vi "ADCP_UI_Event_Structure.vi"(8 "error in (no error)":errorcluster, 11 "ADCU_GUI References":T1) -> ()   [LabVIEW 2017]
uses:
  Controls/ADCP_UI/ADCP_UI_Parameters.ctl
  Controls/ADCP_UI/ADCP_UI_Queues.ctl
  Controls/ADCP_UI/ADCP_UI_Continuous_Receiver_States.ctl
  Controls/ADCP_UI/ADCP_Queue_Receive_Log_Queue_Element.ctl
  Controls/Packet/Packet.ctl
  Controls/Packet/Packet_Direction.ctl
  Controls/Packet/Packet_Type.ctl
  Controls/Packet/Packet_Priority.ctl
  Controls/Data Packets/Data_Packet.ctl
  Controls/Data Packets/Parameter.ctl
  Controls/Data Packets/Parameter_Data_Type.ctl
  Controls/Data Packets/Data_Packet_Transmit_Mode.ctl
  Controls/Data Packets/Data_Packet_FGV_Commands.ctl
  Controls/ADCP_UI/ADCP_UI_Queue_Manager_Commands.ctl
  Controls/Connection Management/Connection_Management_Commands.ctl
  Controls/ADCP_UI/ADCP_UI_Node_Requests.ctl
  ADCP_UI_Receive_List_Data_Packets.vi
panel:
  out "Connect/Disconnect COM Port":bool
  out "Remove transmit list frame":bool
  out "Add transmit list frame":bool
  out "Request frames from node":bool
  out "Add request frame":bool
  out "Remove request frame":bool
  out "Enable / disable node":bool
  out "Get node status":bool
  out "Reset nodes":bool
  out "Reset node":bool
  out "Load Symbol File":bool
  out "Application Stoppped":bool
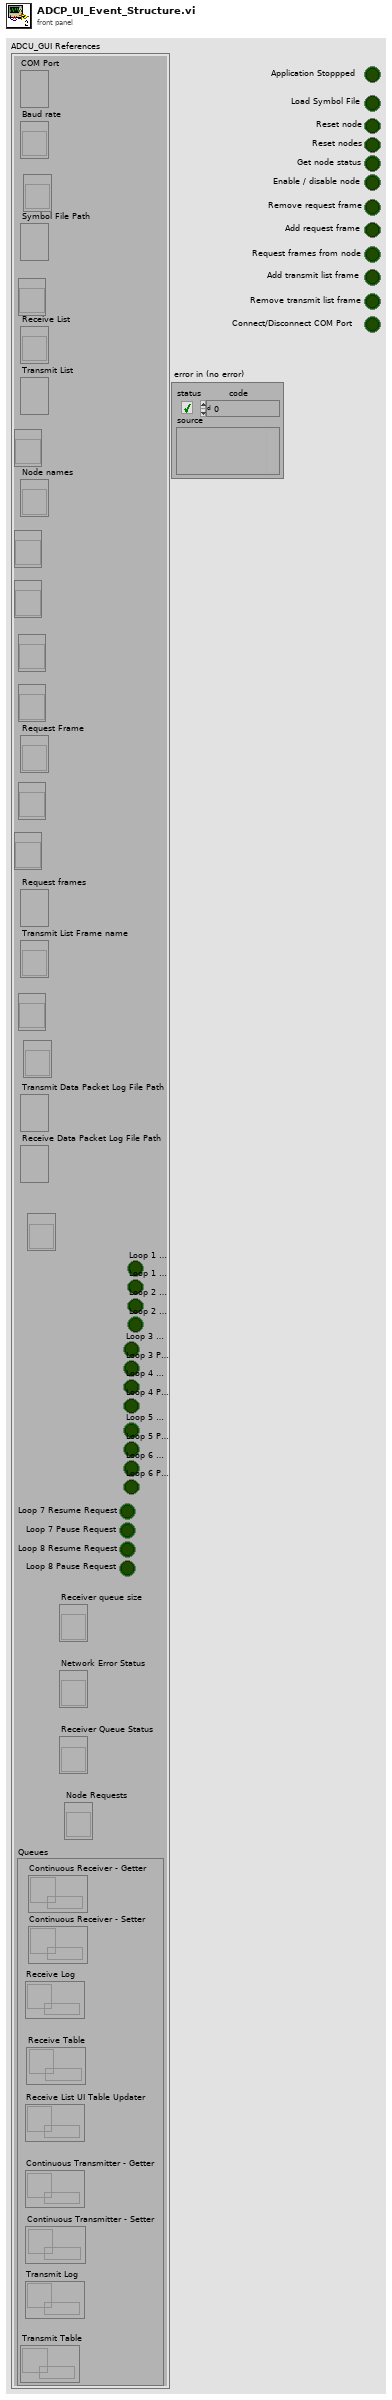
[diagram p1: front panel]
types:
  T1 = typedef "ADCP_UI_Parameters.ctl" = cluster{"COM Port":refnum<vi>, "Baud rate":refnum<vi>, "Symbol File Path":refnum<vi>, "Receive List":refnum<vi>, "Transmit List":refnum<vi>, "Node names":refnum<vi>, "Request Frame":refnum<vi>, "Request frames":refnum<vi>, "Transmit List Frame name":refnum<vi>, "Transmit Data Packet Log File Path":refnum<vi>, "Receive Data Packet Log File Path":refnum<vi>, "Loop 1 Resume Request":bool, "Loop 1 Pause Request":bool, "Loop 2 Resume Request":bool, "Loop 2 Pause Request":bool, "Loop 3 Resume Request":bool, "Loop 3 Pause Request":bool, "Loop 4 Resume Request":bool, "Loop 4 Pause Request":bool, "Loop 5 Resume Request":bool, "Loop 5 Pause Request":bool, "Loop 6 Resume Request":bool, "Loop 6 Pause Request":bool, "Loop 7 Resume Request":bool, "Loop 7 Pause Request":bool, "Loop 8 Resume Request":bool, "Loop 8 Pause Request":bool, "Exit":refnum<vi>, "Connect/Disconnect":refnum<vi>, "Load Symbol File":refnum<vi>, "Reset node":refnum<vi>, "Reset nodes":refnum<vi>, "Get node status":refnum<vi>, "Enable/disable node":refnum<vi>, "Request frames from node":refnum<vi>, "Remove request frame":refnum<vi>, "Add request frame":refnum<vi>, "Remove transmit list frame":refnum<vi>, "Add transmit list frame":refnum<vi>, "Receiver queue size":refnum<vi>, "Network Error Status":refnum<vi>, "Receiver Queue Status":refnum<vi>, "Node Requests":refnum<vi>, "Queues":T2}
  T2 = typedef "ADCP_UI_Queues.ctl" = cluster{"Continuous Receiver - Getter":refnum<queue>, "Continuous Receiver - Setter":refnum<queue>, "Receive Log":refnum<queue>, "Receive Table":refnum<queue>, "Receive List UI Table Updater":refnum<queue>, "Continuous Transmitter - Getter":refnum<queue>, "Continuous Transmitter - Setter":refnum<queue>, "Transmit Log":refnum<queue>, "Transmit Table":refnum<queue>}
  T3 = typedef "Data_Packet_FGV_Commands.ctl" = enum16{"Update all parameters from data packets", "Update Packet", "Load", "Read Packet Parameters", "Write Packet Parameters", "Read Packet Parameter", "Write Packet Parameter", "Read Data Packets", "Read Data Packet", "Read Data Packet by Parameter Name", "Get Parameter Node and Frame ID", "Read Data Packet from Node ID and Frame ID"}
  T4 = typedef "ADCP_UI_Queue_Manager_Commands.ctl" = enum16{"Disable Continuous Receiver", "Enable Continuous Receiver", "Disable Continuous Transmitter", "Enable Continuous Transmitter", "Enable Continuous Tx & Rx", "Disable Continuous Tx & Rx"}
  T5 = typedef "ADCP_UI_Node_Requests.ctl" = enum16{"None", "Open Connection RQST", "Open Connection ACK", "Close Connection RQST", "Close Connection ACK", "Sync/Reset RQST", "Sync/Reset ACK", "Error & Status RQST", "Error & Status ACK", "Remote Request RQST", "Remote Request ACK", "Timeout"}
  T6 = typedef "Connection_Management_Commands.ctl" = enum16{"Sync/Reset", "Open Connection", "Close Connection"}
  T7 = typedef "Packet.ctl" = cluster{"Raw Bytes":u8[], "Checksum":bool, "Direction":T8, "Processed Bytes":u8[], "Node ID":u8, "Packet type":T9, "Frame Data":u32, "Priority":T10, "Frame ID":u8}
  T8 = typedef "Packet_Direction.ctl" = enum16{"Transmit", "Receive", "Bidirectional"}
  T9 = typedef "Packet_Type.ctl" = enum16{"Data", "Connection Management", "Remote Request", "Error/Status"}
  T10 = typedef "Packet_Priority.ctl" = enum16{"LOW", "HIGH"}
  T11 = typedef "Data_Packet_Transmit_Mode.ctl" = enum16{"Disabled", "Single", "Cyclic"}
  T12 = typedef "Parameter.ctl" = cluster{"Parameter name":string, "Node name":string, "Node ID":u8, "Frame name":string, "Frame ID":u8, "Data type":T13, "Start Bit":i32, "Bit Length":i32, "Factor":dbl, "Offset":dbl, "Minimum":dbl, "Maximum":dbl, "Descriptor":string, "Enum values":string[], "Value":string}
  T13 = typedef "Parameter_Data_Type.ctl" = enum16{"BOOL", "UNSIGNED", "SIGNED", "FLOAT32", "ENUM"}
  T14 = typedef "LVComboBoxStrsAndValuesArrayTypeDef.ctl" = cluster{"String":string, "Value":string}[]
  T15 = typedef "CM_Param.ctl" = cluster{"Sync/Reset RQST":bool, "Sync/Reset ACK":bool, "Open Conn. RQST":bool, "Open Conn. ACK":bool, "Close Conn. RQST":bool, "Close Conn. ACK":bool}
  T16 = typedef "ES_Param.ctl" = cluster{"Status Request":bool, "Status Ack.":bool, "Receiver Queue Status":enum16{"OK", "EMPTY", "FULL"}, "Network Error Status":enum16{"NONE", "CONNECTION_ALREADY_OPEN", "CONNECTION_ALREADY_CLOSED", "INVALID_FRAME_REQUEST"}, "Application Error Code":u16, "Receiver Queue Size":i32}
  T17 = enum16{"NONE", "CONNECTION_ALREADY_OPEN", "CONNECTION_ALREADY_CLOSED", "INVALID_FRAME_REQUEST"}
  T18 = typedef "RREQ_Param.ctl" = cluster{"Remote Request":bool, "Remote Ack.":bool, "Number of frames":u8, "FID_0":u8, "FID_1":u8, "FID_2":u8, "FID_3":u8}
  T19 = typedef "ADCP_UI_Data_Packet_Receiver_Parameters.ctl" = cluster{"Node ID":u32, "Frame ID":u32, "Count":u32, "Last received time (ms)":u32, "Time interval (ms)":u32}
  T20 = typedef "Data_Packet.ctl" = cluster{"Packet":T7, "Parameters":T12[], "Last Received Time (ms)":u64, "Receive count":i32, "Transmit count":i32, "Transmit interval (ms)":u32, "Last Transmitted Time (ms)":u64, "Receive interval (ms)":u32, "Transmit_Mode":T11, "Transmit Enable":bool, "Cyclic Transmit interval (ms)":u32}
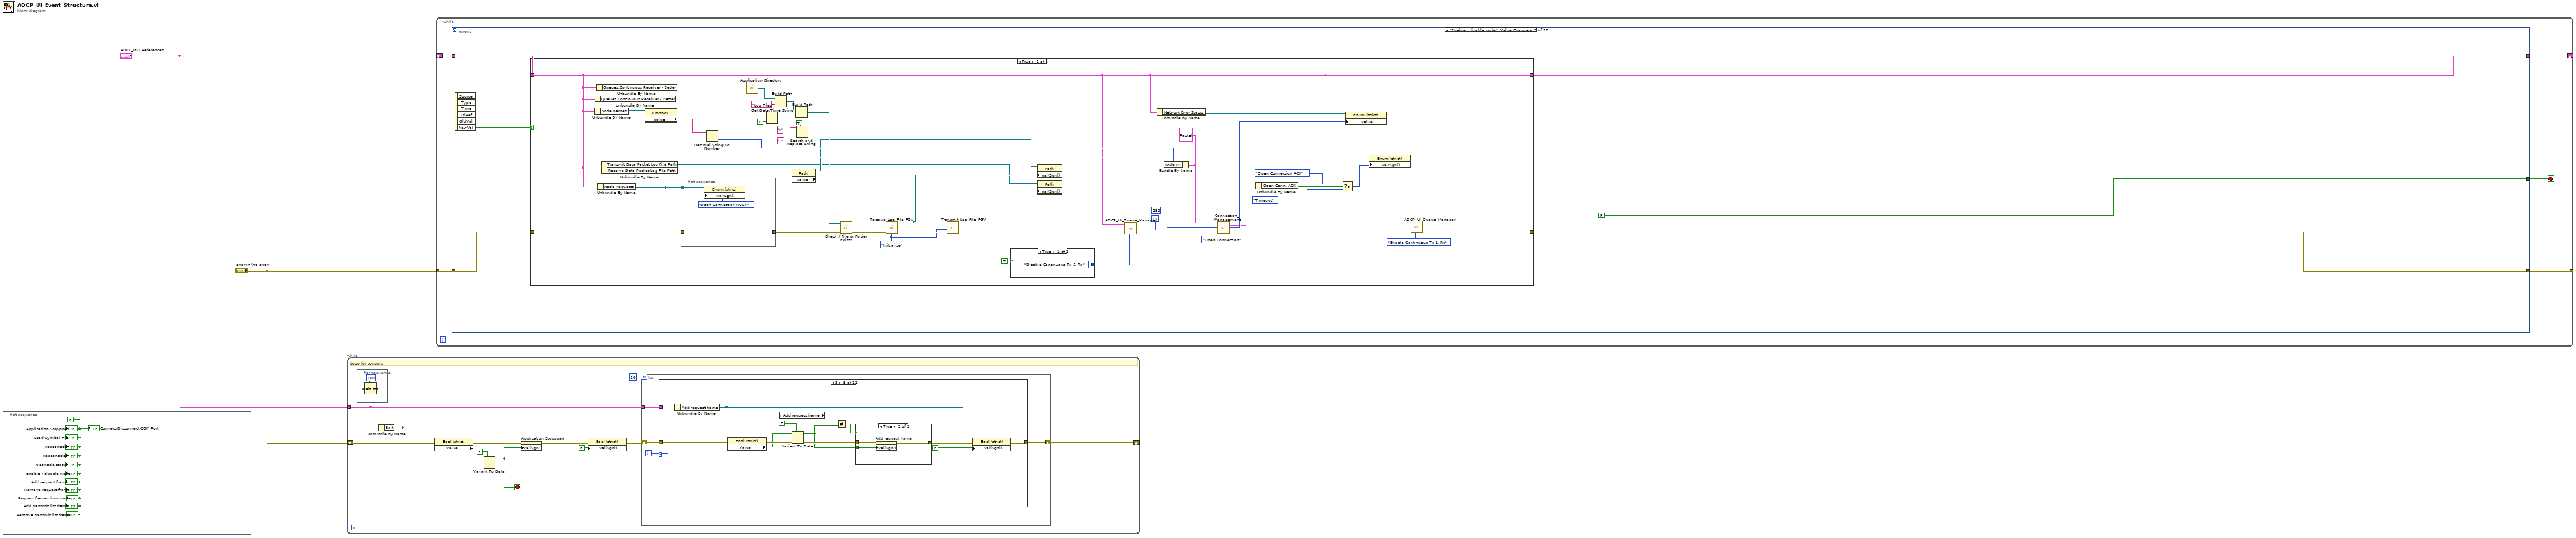
[diagram p0: block diagram]
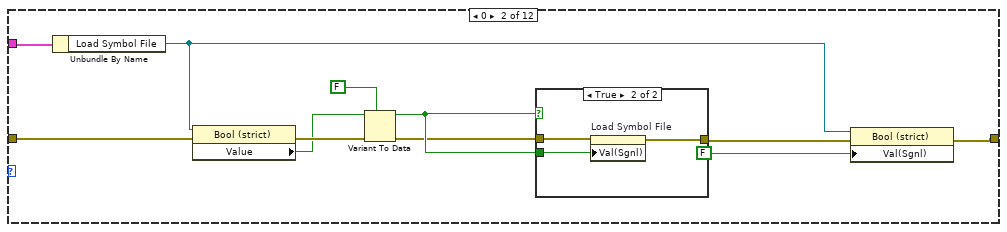
[diagram p3: hidden frame]
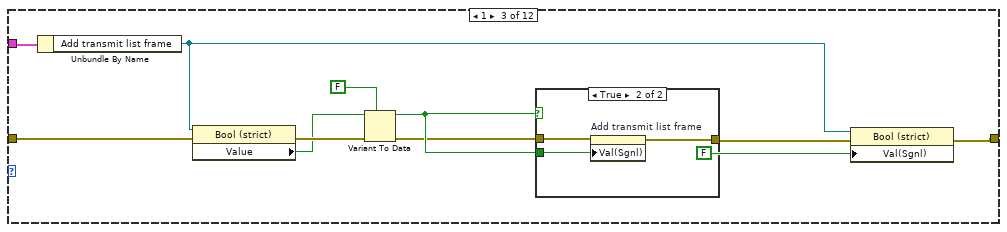
[diagram p5: hidden frame]
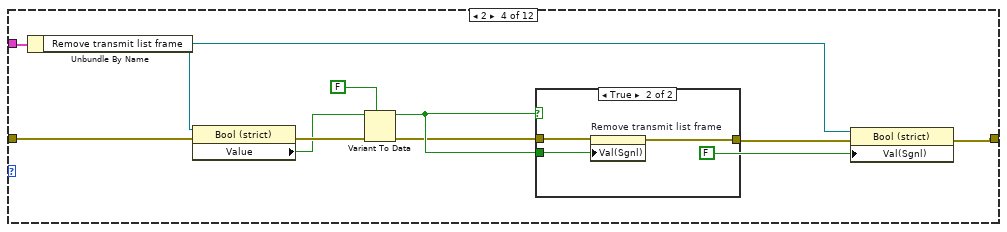
[diagram p7: hidden frame]
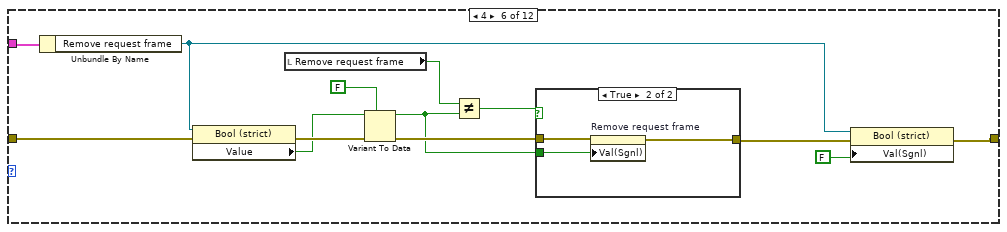
[diagram p10: hidden frame]
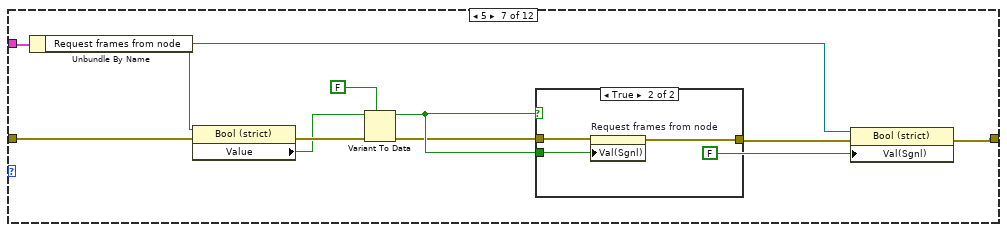
[diagram p12: hidden frame]
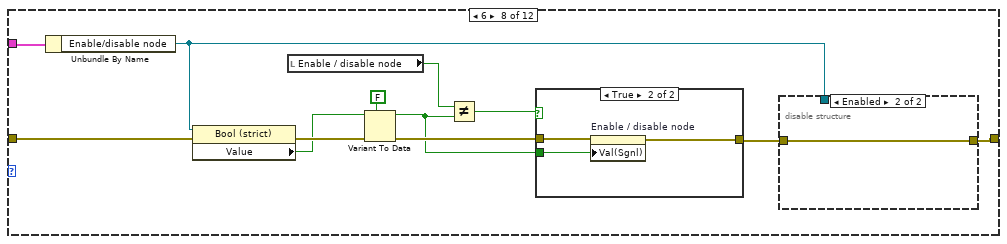
[diagram p14: hidden frame]
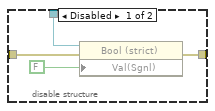
[diagram p15: hidden frame]
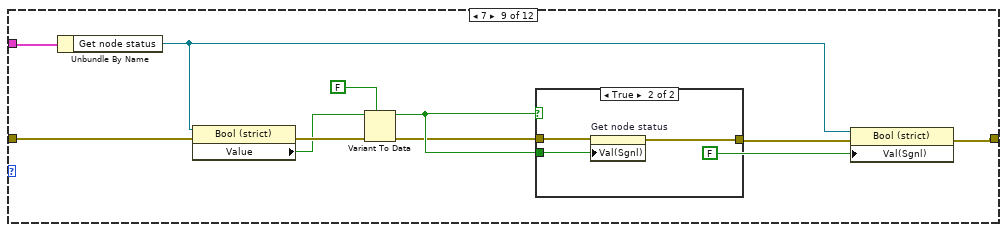
[diagram p17: hidden frame]
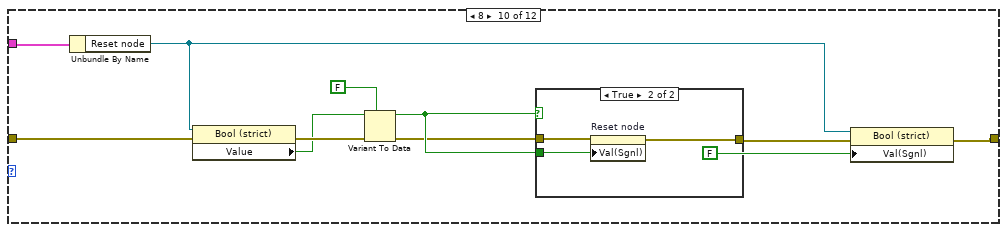
[diagram p19: hidden frame]
diagram:
  n1 = flat-sequence {
    frame #0 {
      w3 = FALSE ("Application Stoppped")
      "Application Stoppped" <- w3
      "Load Symbol File" <- w3
      "Reset node" <- w3
      "Reset nodes" <- w3
      "Get node status" <- w3
      "Enable / disable node" <- w3
      "Add request frame" <- w3
      "Remove request frame" <- w3
      "Request frames from node" <- w3
      "Add transmit list frame" <- w3
      "Remove transmit list frame" <- w3
      "Connect/Disconnect COM Port" <- w3
    }
  }
  n2 = while {
    tunnel: "ADCU_GUI References" -> [w11]
    shift-right: [w9] -> _
    shift-left: "error in (no error)" -> [w13]
    stop <- w14 stop-if-true
    # "Loop for controls"
    n3 = flat-sequence {
      frame #0 {
        n4 = Wait (ms)(milliseconds to wait=u32 100) -> ()  [unwired: 1 out]
      }
    }
    n5 = Unbundle By Name(w11) -> ("Exit"=w6:refnum<vi>)
    n6 = property class="Bool (strict)"(reference=w6, error in=w13) -> (error out=w12:errorcluster, "Value"=w15:bool)  [unwired: 1 out]
    n7 = Variant To Data(type=FALSE, Variant=w15) -> (data=w14:bool)  [unwired: 1 in, 1 out]
    n8 = property on="Application Stoppped" class="Bool (strict)"(error in=w12, "Val(Sgnl)"=w14) -> (error out=w7:errorcluster)  [unwired: 1 in, 1 out]
    n9 = property class="Bool (strict)"(reference=w6, error in=w7, "Val(Sgnl)"=FALSE ("Value (Signaling)")) -> (error out=w5:errorcluster)  [unwired: 1 out]
    n10 = for {
      N: 20 -> [_]
      shift-right: [w17] -> w9
      shift-left: w5 -> [w18]
      tunnel: w11 -> [w16]
      i -> [w19]
      n11 = case shown="3" w19 {
        tunnel: w18 -> [w20 w30 w45 w60 w77 w94 w109 w125 w145 w160 w175 w191]
        tunnel: [w20 w22 w37 w52 w70 w87 w101 w118 w137 w152 w167 w184] -> w17
        tunnel: w16 -> [_ w31 w46 w61 w78 w95 w110 w126 w146 w161 w176 w192]
        frame Default {
        }
        frame 0 {
          n12 = Unbundle By Name(w31) -> ("Load Symbol File"=w23:refnum<vi>)
          n13 = property class="Bool (strict)"(reference=w23, error in=w30) -> (error out=w29:errorcluster, "Value"=w27:bool)  [unwired: 1 out]
          n14 = Variant To Data(error in=w29, type=FALSE, Variant=w27) -> (data=w26:bool, error out=w25:errorcluster)
          n15 = case shown="True" w26 {
            tunnel: w26 -> [_ w35]
            tunnel: [w32 w34] -> w24
            tunnel: w25 -> [w32 w33]
            frame False {
            }
            frame True {
              n16 = property on="Load Symbol File" class="Bool (strict)"(error in=w33, "Val(Sgnl)"=w35) -> (error out=w34:errorcluster)  [unwired: 1 in, 1 out]
            }
          }
          n17 = property class="Bool (strict)"(reference=w23, error in=w24, "Val(Sgnl)"=FALSE) -> (error out=w22:errorcluster)  [unwired: 1 out]
        }
        frame 1 {
          n18 = Unbundle By Name(w46) -> ("Add transmit list frame"=w38:refnum<vi>)
          n19 = property class="Bool (strict)"(reference=w38, error in=w45) -> (error out=w44:errorcluster, "Value"=w42:bool)  [unwired: 1 out]
          n20 = Variant To Data(error in=w44, type=FALSE, Variant=w42) -> (data=w41:bool, error out=w40:errorcluster)
          n21 = case shown="True" w41 {
            tunnel: w41 -> [_ w50]
            tunnel: [w47 w49] -> w39
            tunnel: w40 -> [w47 w48]
            frame False {
            }
            frame True {
              n22 = property on="Add transmit list frame" class="Bool (strict)"(error in=w48, "Val(Sgnl)"=w50) -> (error out=w49:errorcluster)  [unwired: 1 in, 1 out]
            }
          }
          n23 = property class="Bool (strict)"(reference=w38, error in=w39, "Val(Sgnl)"=FALSE) -> (error out=w37:errorcluster)  [unwired: 1 out]
        }
        frame 2 {
          n24 = Unbundle By Name(w61) -> ("Remove transmit list frame"=w53:refnum<vi>)
          n25 = property class="Bool (strict)"(reference=w53, error in=w60) -> (error out=w59:errorcluster, "Value"=w57:bool)  [unwired: 1 out]
          n26 = Variant To Data(error in=w59, type=FALSE, Variant=w57) -> (data=w56:bool, error out=w55:errorcluster)
          n27 = case shown="True" w56 {
            tunnel: w56 -> [_ w65]
            tunnel: [w62 w64] -> w54
            tunnel: w55 -> [w62 w63]
            frame False {
            }
            frame True {
              n28 = property on="Remove transmit list frame" class="Bool (strict)"(error in=w63, "Val(Sgnl)"=w65) -> (error out=w64:errorcluster)  [unwired: 1 in, 1 out]
            }
          }
          n29 = property class="Bool (strict)"(reference=w53, error in=w54, "Val(Sgnl)"=FALSE) -> (error out=w52:errorcluster)  [unwired: 1 out]
        }
        frame 3 {
          n30 = Unbundle By Name(w78) -> ("Add request frame"=w71:refnum<vi>)
          n31 = property class="Bool (strict)"(reference=w71, error in=w77) -> (error out=w76:errorcluster, "Value"=w74:bool)  [unwired: 1 out]
          n32 = local read "Add request frame"() -> (w68:bool)
          n33 = Variant To Data(error in=w76, type=FALSE, Variant=w74) -> (data=w67:bool, error out=w73:errorcluster)
          n34 = Not Equal?(x=w68, y=w67) -> (x != y?=w66:bool)
          n35 = case shown="True" w66 {
            tunnel: w67 -> [_ w82]
            tunnel: [w79 w81] -> w72
            tunnel: w73 -> [w79 w80]
            frame False {
            }
            frame True {
              n36 = property on="Add request frame" class="Bool (strict)"(error in=w80, "Val(Sgnl)"=w82) -> (error out=w81:errorcluster)  [unwired: 1 in, 1 out]
            }
          }
          n37 = property class="Bool (strict)"(reference=w71, error in=w72, "Val(Sgnl)"=FALSE) -> (error out=w70:errorcluster)  [unwired: 1 out]
        }
        frame 4 {
          n38 = Unbundle By Name(w95) -> ("Remove request frame"=w88:refnum<vi>)
          n39 = property class="Bool (strict)"(reference=w88, error in=w94) -> (error out=w93:errorcluster, "Value"=w91:bool)  [unwired: 1 out]
          n40 = local read "Remove request frame"() -> (w83:bool)
          n41 = Variant To Data(error in=w93, type=FALSE, Variant=w91) -> (data=w85:bool, error out=w90:errorcluster)
          n42 = Not Equal?(x=w83, y=w85) -> (x != y?=w84:bool)
          n43 = case shown="True" w84 {
            tunnel: w85 -> [_ w99]
            tunnel: [w96 w98] -> w89
            tunnel: w90 -> [w96 w97]
            frame False {
            }
            frame True {
              n44 = property on="Remove request frame" class="Bool (strict)"(error in=w97, "Val(Sgnl)"=w99) -> (error out=w98:errorcluster)  [unwired: 1 in, 1 out]
            }
          }
          n45 = property class="Bool (strict)"(reference=w88, error in=w89, "Val(Sgnl)"=FALSE) -> (error out=w87:errorcluster)  [unwired: 1 out]
        }
        frame 5 {
          n46 = Unbundle By Name(w110) -> ("Request frames from node"=w102:refnum<vi>)
          n47 = property class="Bool (strict)"(reference=w102, error in=w109) -> (error out=w108:errorcluster, "Value"=w106:bool)  [unwired: 1 out]
          n48 = Variant To Data(error in=w108, type=FALSE, Variant=w106) -> (data=w105:bool, error out=w104:errorcluster)
          n49 = case shown="True" w105 {
            tunnel: w105 -> [_ w114]
            tunnel: [w111 w113] -> w103
            tunnel: w104 -> [w111 w112]
            frame False {
            }
            frame True {
              n50 = property on="Request frames from node" class="Bool (strict)"(error in=w112, "Val(Sgnl)"=w114) -> (error out=w113:errorcluster)  [unwired: 1 in, 1 out]
            }
          }
          n51 = property class="Bool (strict)"(reference=w102, error in=w103, "Val(Sgnl)"=FALSE) -> (error out=w101:errorcluster)  [unwired: 1 out]
        }
        frame 6 {
          n52 = Unbundle By Name(w126) -> ("Enable/disable node"=w119:refnum<vi>)
          n53 = property class="Bool (strict)"(reference=w119, error in=w125) -> (error out=w124:errorcluster, "Value"=w122:bool)  [unwired: 1 out]
          n54 = local read "Enable / disable node"() -> (w115:bool)
          n55 = Variant To Data(error in=w124, type=FALSE, Variant=w122) -> (data=w116:bool, error out=w121:errorcluster)
          n56 = Not Equal?(x=w115, y=w116) -> (x != y?=w117:bool)
          n57 = case shown="True" w117 {
            tunnel: w116 -> [_ w135]
            tunnel: [w132 w134] -> w120
            tunnel: w121 -> [w132 w133]
            frame False {
            }
            frame True {
              n58 = property on="Enable / disable node" class="Bool (strict)"(error in=w133, "Val(Sgnl)"=w135) -> (error out=w134:errorcluster)  [unwired: 1 in, 1 out]
            }
          }
          n59 = disable-structure shown="Enabled" {
            disable-tunnel: w120 -> [w130 w131]
            disable-tunnel: w119 -> [w129 _]
            disable-tunnel: [w128 w131] -> w118
            frame Disabled {
              n60 = property class="Bool (strict)"(reference=w129, error in=w130, "Val(Sgnl)"=FALSE) -> (error out=w128:errorcluster)  [unwired: 1 out]
            }
            frame Enabled {
            }
          }
        }
        frame 7 {
          n61 = Unbundle By Name(w146) -> ("Get node status"=w138:refnum<vi>)
          n62 = property class="Bool (strict)"(reference=w138, error in=w145) -> (error out=w144:errorcluster, "Value"=w142:bool)  [unwired: 1 out]
          n63 = Variant To Data(error in=w144, type=FALSE, Variant=w142) -> (data=w141:bool, error out=w140:errorcluster)
          n64 = case shown="True" w141 {
            tunnel: w141 -> [_ w150]
            tunnel: [w147 w149] -> w139
            tunnel: w140 -> [w147 w148]
            frame False {
            }
            frame True {
              n65 = property on="Get node status" class="Bool (strict)"(error in=w148, "Val(Sgnl)"=w150) -> (error out=w149:errorcluster)  [unwired: 1 in, 1 out]
            }
          }
          n66 = property class="Bool (strict)"(reference=w138, error in=w139, "Val(Sgnl)"=FALSE) -> (error out=w137:errorcluster)  [unwired: 1 out]
        }
        frame 8 {
          n67 = Unbundle By Name(w161) -> ("Reset node"=w153:refnum<vi>)
          n68 = property class="Bool (strict)"(reference=w153, error in=w160) -> (error out=w159:errorcluster, "Value"=w157:bool)  [unwired: 1 out]
          n69 = Variant To Data(error in=w159, type=FALSE, Variant=w157) -> (data=w156:bool, error out=w155:errorcluster)
          n70 = case shown="True" w156 {
            tunnel: w156 -> [_ w165]
            tunnel: [w162 w164] -> w154
            tunnel: w155 -> [w162 w163]
            frame False {
            }
            frame True {
              n71 = property on="Reset node" class="Bool (strict)"(error in=w163, "Val(Sgnl)"=w165) -> (error out=w164:errorcluster)  [unwired: 1 in, 1 out]
            }
          }
          n72 = property class="Bool (strict)"(reference=w153, error in=w154, "Val(Sgnl)"=FALSE) -> (error out=w152:errorcluster)  [unwired: 1 out]
        }
        frame 9 {
          n73 = Unbundle By Name(w176) -> ("Reset nodes"=w168:refnum<vi>)
          n74 = property class="Bool (strict)"(reference=w168, error in=w175) -> (error out=w174:errorcluster, "Value"=w172:bool)  [unwired: 1 out]
          n75 = Variant To Data(error in=w174, type=FALSE, Variant=w172) -> (data=w171:bool, error out=w170:errorcluster)
          n76 = case shown="True" w171 {
            tunnel: w171 -> [_ w180]
            tunnel: [w177 w179] -> w169
            tunnel: w170 -> [w177 w178]
            frame False {
            }
            frame True {
              n77 = property on="Reset nodes" class="Bool (strict)"(error in=w178, "Val(Sgnl)"=w180) -> (error out=w179:errorcluster)  [unwired: 1 in, 1 out]
            }
          }
          n78 = property class="Bool (strict)"(reference=w168, error in=w169, "Val(Sgnl)"=FALSE) -> (error out=w167:errorcluster)  [unwired: 1 out]
        }
        frame 10 {
          n79 = Unbundle By Name(w192) -> ("Connect/Disconnect"=w185:refnum<vi>)
          n80 = property class="Bool (strict)"(reference=w185, error in=w191) -> (error out=w190:errorcluster, "Value"=w188:bool)  [unwired: 1 out]
          n81 = local read "Connect/Disconnect COM Port"() -> (w181:bool)
          n82 = Variant To Data(error in=w190, type=FALSE, Variant=w188) -> (data=w182:bool, error out=w187:errorcluster)
          n83 = Not Equal?(x=w181, y=w182) -> (x != y?=w183:bool)
          n84 = case shown="True" w183 {
            tunnel: w182 -> [_ w201]
            tunnel: [w198 w200] -> w186
            tunnel: w187 -> [w198 w199]
            frame False {
            }
            frame True {
              n85 = property on="Connect/Disconnect COM Port" class="Bool (strict)"(error in=w199, "Val(Sgnl)"=w201) -> (error out=w200:errorcluster)  [unwired: 1 in, 1 out]
            }
          }
          n86 = disable-structure shown="Enabled" {
            disable-tunnel: w186 -> [w196 w197]
            disable-tunnel: w185 -> [w195 _]
            disable-tunnel: [w194 w197] -> w184
            frame Disabled {
              n87 = property class="Bool (strict)"(reference=w195, error in=w196, "Val(Sgnl)"=FALSE) -> (error out=w194:errorcluster)  [unwired: 1 out]
            }
            frame Enabled {
            }
          }
        }
      }
    }
  }
  n88 = while {
    tunnel: "error in (no error)" -> [w207]
    shift-right: [w204] -> _
    shift-left: "ADCU_GUI References" -> [w205]
    tunnel: [w203] -> _
    stop <- w206 stop-if-true
    n89 = event shown="[8] \"Enable / disable node\": Value Change" {
      selector: _ -> [_ _ _ _ _ _ _ _ _ _ _ _]
      dyn-events: _ -> [_ _ _ _ _ _ _ _ _ _ _ _]
      timeout: _ -> [_ _ _ _ _ _ _ _ _ _ _ _]
      tunnel: w207 -> [w208 w213 w239 w281 w294 w330 w365 w404 w449 w532 w625 w670]
      tunnel: [FALSE w214 FALSE ("NewVal") FALSE ("NewVal") FALSE ("NewVal") FALSE ("NewVal") FALSE ("NewVal") FALSE ("NewVal") FALSE ("NewVal") FALSE ("NewVal") FALSE ("NewVal") FALSE ("NewVal")] -> w206
      tunnel: w205 -> [w210 w215 w222 w272 w292 w328 w363 w402 w447 w530 w622 w667]
      tunnel: [w210 w215 w222 w272 w291 w327 w362 w401 w446 w529 w621 w666] -> w204
      tunnel: [w208 w213 w236 w273 w293 w329 w364 w403 w448 w531 w623 w668] -> w203
      event Timeout {
        n90 = event-data() -> ()  [unwired: 1 in, 3 out]
      }
      event "Application Stoppped": Value Change {
        n91 = event-data() -> ("CtlRef"=w212:refnum<vi>, "NewVal"=w214:bool)  [unwired: 1 in, 4 out]
        n92 = property class="Bool (strict)"(reference=w212, "Val(Sgnl)"=FALSE ("Value")) -> ()  [unwired: 1 in, 2 out]
      }
      event "Load Symbol File": Value Change {
        n93 = event-data() -> ()  [unwired: 1 in, 6 out]
        n94 = Unbundle By Name(w222) -> ("Symbol File Path"=w240:refnum<vi>)
        n95 = Unbundle By Name(w222) -> ("Load Symbol File"=w234:refnum<vi>)
        n96 = property class="Path"(reference=w240, error in=w239) -> (error out=w238:errorcluster, "Value"=w237:path)  [unwired: 1 out]
        n97 = property class="Bool (strict)"(reference=w234, "Val(Sgnl)"=FALSE ("Value (Signaling)")) -> ()  [unwired: 1 in, 2 out]
        n98 = call "Data_Packet_FGV.vi"("Symbol File Path"=w237, "error in (no error)"=w238, "Commands"=Data_Packet_FGV_Commands."Load") -> ("Parameters out"=w232:T12[], "error out"=w236:errorcluster)  [unwired: 7 in, 4 out]
        n99 = for {
          tunnel: w232 -> [w265] mode=indexing
          tunnel: [w267] -> w231 mode=indexing
          tunnel: [w268] -> w228 mode=indexing
          tunnel: [w266] -> w217 mode=indexing
          tunnel: [w264] -> w219 mode=indexing
          n100 = Unbundle By Name(w265) -> ("Node name"=w267:string)
          n101 = Unbundle By Name(w265) -> ("Frame name"=w270:string)
          n102 = Unbundle By Name(w265) -> ("Frame ID"=w264:u8)
          n103 = Unbundle By Name(w265) -> ("Node ID"=w266:u8)
          n104 = Concatenate Strings(w267, ":" ("string"), w270) -> (w268:string)
        }
        n105 = for {
          tunnel: w231 -> [w262] mode=indexing
          shift-right: [w261] -> _
          shift-left: "" -> [w263]
          tunnel: [w261] -> w226 mode=indexing if=w258
          tunnel: [w259] -> w216 mode=indexing if=w258
          tunnel: w217 -> [w259] mode=indexing
          n106 = Equal?(x=w263, y=w262) -> (x = y?=w260:bool)
          n107 = Select(t=w263, s=w260, f=w262) -> (s? t:f=w261:string)
          n108 = Not(x=w260) -> (.not. x?=w258:bool)
        }
        n109 = for {
          tunnel: w228 -> [w256] mode=indexing
          shift-right: [w255] -> _
          shift-left: "" -> [w257]
          tunnel: [w255] -> w224 mode=indexing if=w252
          tunnel: w219 -> [w253] mode=indexing
          tunnel: [w253] -> w218 mode=indexing if=w252
          n110 = Equal?(x=w257, y=w256) -> (x = y?=w254:bool)
          n111 = Select(t=w257, s=w254, f=w256) -> (s? t:f=w255:string)
          n112 = Not(x=w254) -> (.not. x?=w252:bool)
        }
        n113 = Unbundle By Name(w222) -> ("Node names"=w227:refnum<vi>, "Request Frame"=w223:refnum<vi>)
        n114 = Unbundle By Name(w222) -> ("Transmit List Frame name"=w221:refnum<vi>)
        n115 = for {
          tunnel: w226 -> [w250] mode=indexing
          tunnel: [w248] -> w225 mode=indexing
          tunnel: w216 -> [w247] mode=indexing
          n116 = Number To Decimal String(number=w247) -> (decimal integer string=w249:string)  [unwired: 1 in]
          n117 = Bundle By Name(cluster=cluster{"String":string, "Value":string} {"String"="", "Value"=""}, "String"=w250, "Value"=w249) -> (w248:cluster{"String":string, "Value":string})
        }
        n118 = for {
          tunnel: w224 -> [w245] mode=indexing
          tunnel: [w243] -> w220 mode=indexing
          tunnel: w218 -> [w242] mode=indexing
          n119 = Number To Decimal String(number=w242) -> (decimal integer string=w244:string)  [unwired: 1 in]
          n120 = Bundle By Name(cluster=cluster{"String":string, "Value":string} {"String"="", "Value"=""}, "String"=w245, "Value"=w244) -> (w243:cluster{"String":string, "Value":string})
        }
        n121 = property class="CmbBox"(reference=w227, "Strings And Values[]"=w225) -> ()  [unwired: 1 in, 2 out]
        n122 = property class="CmbBox"(reference=w223, "Strings And Values[]"=w220) -> ()  [unwired: 1 in, 2 out]
        n123 = property class="CmbBox"(reference=w221, "Strings And Values[]"=w220) -> ()  [unwired: 1 in, 2 out]
      }
      event "Connect/Disconnect COM Port": Value Change {
        n124 = event-data() -> ()  [unwired: 1 in, 6 out]
        n125 = Unbundle By Name(w272) -> ("COM Port"=w280:refnum<vi>, "Baud rate"=w278:refnum<vi>)
        n126 = property class="DigNum (strict)"(reference=w278) -> ("Value"=w277:u32)  [unwired: 1 in, 2 out]
        n127 = property class="VISAName"(reference=w280) -> ("Value"=w279:refnum<visa-resource-name>)  [unwired: 1 in, 2 out]
        n128 = call "Serial_Port_FGV.vi"("error in (no error)"=w281, "Initialize ?"=TRUE, "baud rate"=w277, "COM Port In"=w279) -> ("error out"=w274:errorcluster)  [unwired: 6 in, 1 out]
        n129 = case shown="True" TRUE {
          tunnel: w274 -> [w282 w285]
          tunnel: [w282 w284] -> w273
          tunnel: w272 -> [_ w283]
          frame False {
          }
          frame True {
            n130 = disable-structure shown="Enabled" {
              disable-tunnel: w285 -> [w289 w290]
              disable-tunnel: [w288 w290] -> w284
              disable-tunnel: w283 -> [w286 _]
              frame Enabled {
                n131 = call "ADCP_UI_Queue_Manager.vi"("error in (no error)"=w289, "command"=ADCP_UI_Queue_Manager_Commands."Enable Continuous Transmitter", "ADCU_GUI References"=w286) -> ("error out"=w288:errorcluster)  [unwired: 8 in]
              }
              frame Disabled {
              }
            }
          }
        }
      }
      event "Add request frame": Value Change {
        n132 = event-data() -> ("NewVal"=w295:bool)  [unwired: 1 in, 5 out]
        n133 = case shown="True" w295 {
          tunnel: w294 -> [w298 w313]
          tunnel: [w298 w305] -> w293
          tunnel: w292 -> [w297 w304]
          tunnel: [w297 w304] -> w291
          frame False {
          }
          frame True {
            n134 = Unbundle By Name(w304) -> ("Request frames"=w312:refnum<vi>)
            n135 = Unbundle By Name(w304) -> ("Request Frame"=w314:refnum<vi>)
            n136 = property class="Arr (strict)"(reference=w312) -> (reference out=w307:refnum<vi>, "Value"=w308:string[])  [unwired: 1 in, 1 out]
            n137 = property class="CmbBox"(reference=w314, error in=w313) -> (error out=w309:errorcluster, "Value"=w301:string, "Strings And Values[]"=w302:T14)  [unwired: 1 out]
            n138 = for {
              tunnel: w302 -> [w319] mode=indexing
              tunnel: w301 -> [w318]
              tunnel: [w315] -> w300
              stop <- w316 stop-if-true
              n139 = Unbundle By Name(w319) -> ("Value"=w317:string, "String"=w315:string)
              n140 = Equal?(x=w318, y=w317) -> (x = y?=w316:bool)
            }
            n141 = Search 1D Array(1D array=w308, element=w300) -> (index of element=w303:i32)  [unwired: 1 in]
            n142 = Equal?(x=w303, y=-1) -> (x = y?=w310:bool)
            n143 = case shown="False" w310 {
              tunnel: w309 -> [w321 w323]
              tunnel: w308 -> [w320 w325]
              tunnel: w300 -> [_ w322]
              tunnel: [w320 w324] -> w299
              tunnel: [w321 w323] -> w306
              tunnel: w302 -> [_ _]
              tunnel: w303 -> [_ _]
              frame False {
              }
              frame True {
                n144 = Build Array (concatenate)(w325, w322) -> (w324:string[])
              }
            }
            n145 = property class="Arr (strict)"(reference=w307, error in=w306, "Value"=w299) -> (error out=w305:errorcluster)  [unwired: 1 out]
          }
        }
      }
      event "Remove request frame": Value Change {
        n146 = event-data() -> ("NewVal"=w326:bool)  [unwired: 1 in, 5 out]
        n147 = case shown="True" w326 {
          tunnel: w330 -> [w333 w348]
          tunnel: [w333 w339] -> w329
          tunnel: w328 -> [w332 w338]
          tunnel: [w332 w338] -> w327
          frame False {
          }
          frame True {
            n148 = Unbundle By Name(w338) -> ("Request frames"=w347:refnum<vi>)
            n149 = Unbundle By Name(w338) -> ("Request Frame"=w349:refnum<vi>)
            n150 = property class="Arr (strict)"(reference=w347) -> (reference out=w342:refnum<vi>, "Value"=w343:string[])  [unwired: 1 in, 1 out]
            n151 = property class="CmbBox"(reference=w349, error in=w348) -> (error out=w344:errorcluster, "Value"=w335:string, "Strings And Values[]"=w336:T14)  [unwired: 1 out]
            n152 = for {
              tunnel: w336 -> [w354] mode=indexing
              tunnel: w335 -> [w352]
              tunnel: [w350] -> w334
              stop <- w351 stop-if-true
              n153 = Unbundle By Name(w354) -> ("Value"=w353:string, "String"=w350:string)
              n154 = Equal?(x=w352, y=w353) -> (x = y?=w351:bool)
            }
            n155 = Search 1D Array(1D array=w343, element=w334) -> (index of element=w337:i32)  [unwired: 1 in]
            n156 = Not Equal?(x=w337, y=-1) -> (x != y?=w345:bool)
            n157 = case shown="True" w345 {
              tunnel: w344 -> [w355 w361]
              tunnel: w343 -> [w356 w360]
              tunnel: w334 -> [_ _]
              tunnel: [w356 w359] -> w341
              tunnel: [w355 w361] -> w340
              tunnel: w337 -> [_ w357]
              frame False {
              }
              frame True {
                n158 = Delete From Array(array=w360, length=1, index=w357) -> (array with subset deleted=w359:string[])  [unwired: 1 out]
              }
            }
            n159 = property class="Arr (strict)"(reference=w342, error in=w340, "Value"=w341) -> (error out=w339:errorcluster)  [unwired: 1 out]
          }
        }
      }
      event "Reset node": Value Change {
        n160 = event-data() -> ("NewVal"=w366:bool)  [unwired: 1 in, 5 out]
        n161 = case shown="True" w366 {
          tunnel: w365 -> [w368 w385]
          tunnel: [w368 w374] -> w364
          tunnel: w363 -> [w369 w371]
          tunnel: [w369 w371] -> w362
          frame False {
          }
          frame True {
            n162 = Unbundle By Name(w371) -> ("Node names"=w393:refnum<vi>)
            n163 = Unbundle By Name(w371) -> ("Node Requests"=w384:refnum<vi>)
            n164 = property class="CmbBox"(reference=w393) -> ("Value"=w392:string)  [unwired: 1 in, 2 out]
            n165 = flat-sequence {
              tunnel: w385 -> [w400]
              tunnel: [w400] -> w377
              tunnel: w384 -> [w399]
              frame #0 {
                n166 = property class="Enum (strict)"(reference=w399, "Val(Sgnl)"=ADCP_UI_Node_Requests."Sync/Reset RQST" ("Value")) -> ()  [unwired: 1 in, 2 out]
              }
            }
            n167 = Decimal String To Number(string=w392) -> (number=w390:i32)  [unwired: 2 in, 1 out]
            n168 = call "ADCP_UI_Queue_Manager.vi"("error in (no error)"=w377, "command"=ADCP_UI_Queue_Manager_Commands."Disable Continuous Tx & Rx", "ADCU_GUI References"=w371) -> ("error out"=w376:errorcluster)  [unwired: 8 in]
            n169 = Bundle By Name(cluster=T7 {"Raw Bytes"=[], "Checksum"=FALSE, "Direction"=enum."Transmit", "Processed Bytes"=[], "Node ID"=0, "Packet type"=enum."Data", "Frame Data"=0, "Priority"=enum."LOW", "Frame ID"=0} ("CM Packet In"), "Node ID"=w390) -> (w389:T7)
            n170 = call "Connection_Management.vi"("CM Packet In"=w389, "Commands"=Connection_Management_Commands."Sync/Reset", "Retry interval (ms)"=250, "Number of tries"=u8 10, "error in (no error)"=w376) -> ("CM Params Out"=w383:T15, "error out"=w373:errorcluster)  [unwired: 7 in, 2 out]
            n171 = Unbundle By Name(w383) -> ("Sync/Reset ACK"=w382:bool)
            n172 = Unbundle By Name(w371) -> ("Node Requests"=w379:refnum<vi>)
            n173 = Select(t=ADCP_UI_Node_Requests."Sync/Reset ACK" ("Value"), s=w382, f=ADCP_UI_Node_Requests."Timeout" ("Value")) -> (s? t:f=w378:T5)
            n174 = property class="Enum (strict)"(reference=w379, "Val(Sgnl)"=w378) -> ()  [unwired: 1 in, 2 out]
            n175 = call "ADCP_UI_Queue_Manager.vi"("error in (no error)"=w373, "command"=ADCP_UI_Queue_Manager_Commands."Enable Continuous Transmitter", "ADCU_GUI References"=w371) -> ("error out"=w372:errorcluster)  [unwired: 8 in]
            n176 = disable-structure shown="Enabled" {
              disable-tunnel: w372 -> [w396 w397]
              disable-tunnel: [w395 w397] -> w374
              disable-tunnel: w371 -> [w394 _]
              frame Disabled {
                n177 = call "ADCP_UI_Queue_Manager.vi"("error in (no error)"=w396, "ADCU_GUI References"=w394) -> ("error out"=w395:errorcluster)  [unwired: 9 in]
              }
              frame Enabled {
              }
            }
          }
        }
      }
      event "Get node status": Value Change {
        n178 = event-data() -> ("NewVal"=w405:bool)  [unwired: 1 in, 5 out]
        n179 = case shown="True" w405 {
          tunnel: w404 -> [w407 w421]
          tunnel: [w407 w411] -> w403
          tunnel: w402 -> [w408 w410]
          tunnel: [w408 w410] -> w401
          frame False {
          }
          frame True {
            n180 = Unbundle By Name(w410) -> ("Node names"=w442:refnum<vi>)
            n181 = Unbundle By Name(w410) -> ("Node Requests"=w428:refnum<vi>)
            n182 = call "ADCP_UI_Queue_Manager.vi"("error in (no error)"=w421, "command"=ADCP_UI_Queue_Manager_Commands."Disable Continuous Tx & Rx", "ADCU_GUI References"=w410) -> ("error out"=w420:errorcluster)  [unwired: 8 in]
            n183 = property class="CmbBox"(reference=w442) -> ("Value"=w441:string)  [unwired: 1 in, 2 out]
            n184 = flat-sequence {
              tunnel: w420 -> [w445]
              tunnel: [w445] -> w429
              tunnel: w428 -> [w444]
              frame #0 {
                n185 = property class="Enum (strict)"(reference=w444, "Val(Sgnl)"=ADCP_UI_Node_Requests."Error & Status RQST" ("Value (Signaling)")) -> ()  [unwired: 1 in, 2 out]
              }
            }
            n186 = Decimal String To Number(string=w441) -> (number=w439:i32)  [unwired: 2 in, 1 out]
            n187 = Unbundle By Name(w410) -> ("Receiver Queue Status"=w435:refnum<vi>)
            n188 = Unbundle By Name(w410) -> ("Network Error Status"=w433:refnum<vi>)
            n189 = Unbundle By Name(w410) -> ("Receiver queue size"=w431:refnum<vi>)
            n190 = Unbundle By Name(w410) -> ("Node Requests"=w423:refnum<vi>)
            n191 = Bundle By Name(cluster=T7 {"Raw Bytes"=[], "Checksum"=FALSE, "Direction"=enum."Transmit", "Processed Bytes"=[], "Node ID"=0, "Packet type"=enum."Data", "Frame Data"=0, "Priority"=enum."LOW", "Frame ID"=0} ("CM Packet In"), "Node ID"=w439) -> (w436:T7)
            n192 = call "Error_and_Status.vi"("error in (no error)"=w429, "Retry interval (ms)"=250, "Number of tries"=u8 10, "ES Packet"=w436) -> ("error out"=w418:errorcluster, "ES Param Out"=w427:T16)  [unwired: 5 in, 1 out]
            n193 = Unbundle By Name(w427) -> ("Receiver Queue Status"=w434:enum16{"OK", "EMPTY", "FULL"}, "Network Error Status"=w432:T17, "Receiver Queue Size"=w430:i32)
            n194 = Unbundle By Name(w427) -> ("Status Ack."=w426:bool)
            n195 = Select(t=ADCP_UI_Node_Requests."Error & Status ACK" ("Enum"), s=w426, f=ADCP_UI_Node_Requests."Timeout" ("Value")) -> (s? t:f=w422:T5)
            n196 = property class="DigNum (strict)"(reference=w431, "Value"=w430) -> ()  [unwired: 1 in, 2 out]
            n197 = property class="Enum (strict)"(reference=w433, "Value"=w432) -> ()  [unwired: 1 in, 2 out]
            n198 = property class="Enum (strict)"(reference=w423, "Val(Sgnl)"=w422) -> ()  [unwired: 1 in, 2 out]
            n199 = property class="Enum (strict)"(reference=w435, "Value"=w434) -> ()  [unwired: 1 in, 2 out]
            n200 = Unbundle By Name(w410) -> ("Enable/disable node"=w414:refnum<vi>)
            n201 = property class="Bool (strict)"(reference=w414) -> ("Value"=w413:bool)  [unwired: 1 in, 2 out]
            n202 = Select(t=ADCP_UI_Queue_Manager_Commands."Enable Continuous Receiver" ("command"), s=w413, f=ADCP_UI_Queue_Manager_Commands."Disable Continuous Receiver" ("command")) -> (s? t:f=w416:T4)
            n203 = call "ADCP_UI_Queue_Manager.vi"("error in (no error)"=w418, "command"=w416, "ADCU_GUI References"=w410) -> ("error out"=w412:errorcluster)  [unwired: 8 in]
            n204 = call "ADCP_UI_Queue_Manager.vi"("error in (no error)"=w412, "command"=ADCP_UI_Queue_Manager_Commands."Enable Continuous Transmitter", "ADCU_GUI References"=w410) -> ("error out"=w411:errorcluster)  [unwired: 8 in]
          }
        }
      }
      event "Enable / disable node": Value Change {
        n205 = event-data() -> ("NewVal"=w450:bool)  [unwired: 1 in, 5 out]
        n206 = case shown="True" w450 {
          tunnel: w449 -> [w485 w514]
          tunnel: [w475 w503] -> w448
          tunnel: w447 -> [w462 w502]
          tunnel: [w462 w502] -> w446
          frame True {
            w454 = enum16{"Initialize", "Update", "Stop"}."Initialize" ("Command")
            w490 = T7 {"Raw Bytes"=[], "Checksum"=FALSE, "Direction"=enum."Transmit", "Processed Bytes"=[], "Node ID"=0, "Packet type"=enum."Data", "Frame Data"=0, "Priority"=enum."LOW", "Frame ID"=0} ("CM Packet In")
            n207 = Unbundle By Name(w462) -> ("Node names"=w494:refnum<vi>)
            n208 = Unbundle By Name(w462) -> ()  [unwired: 1 out]
            n209 = Unbundle By Name(w462) -> ()  [unwired: 1 out]
            n210 = Unbundle By Name(w462) -> ("Node Requests"=w484:refnum<vi>)
            n211 = Unbundle By Name(w462) -> ("Transmit Data Packet Log File Path"=w453:refnum<vi>, "Receive Data Packet Log File Path"=w461:refnum<vi>)
            n212 = property class="CmbBox"(reference=w494) -> ("Value"=w493:string)  [unwired: 1 in, 2 out]
            n213 = flat-sequence {
              tunnel: w485 -> [w499]
              tunnel: [w499] -> w469
              tunnel: w484 -> [w498]
              frame #0 {
                n214 = property class="Enum (strict)"(reference=w498, "Val(Sgnl)"=ADCP_UI_Node_Requests."Open Connection RQST" ("Value (Signaling)")) -> ()  [unwired: 1 in, 2 out]
              }
            }
            n215 = Decimal String To Number(string=w493) -> (number=w492:i32)  [unwired: 2 in, 1 out]
            n216 = call <vilib>:"Application Directory.vi"() -> ("Application Directory"=w473:path)
            n217 = Get Date/Time String(want seconds? (F)=TRUE) -> (date string=w470:string, time string=w466:string)  [unwired: 2 in]
            n218 = Build Path(base path=w473, name or relative path="Log Files") -> (appended path=w471:path)
            n219 = property class="Path" props=["Value"](reference=w461) -> (reference out=w460:refnum<vi>)  [unwired: 1 in, 2 out]
            n220 = Build Path(base path=w471, name or relative path=w470) -> (appended path=w468:path)
            n221 = Search and Replace String(replace all?=TRUE ("replace all? (F)"), input string=w466, search string=":", replace string="_" ("replace string (\"\")")) -> ()  [unwired: 4 in, 4 out]
            n222 = call <vilib>:"Check if File or Folder Exists.vi"("error in (no error)"=w469, "path"=w468) -> ("error out"=w458:errorcluster)  [unwired: 7 in, 2 out]
            n223 = call "Receive_Log_File_FGV.vi"("error in (no error)"=w458, "Command"=w454) -> ("error out"=w456:errorcluster, "Receive Log File Path"=w457:path)  [unwired: 8 in]
            n224 = call "Transmit_Log_File_FGV.vi"("error in (no error)"=w456, "Command"=w454) -> ("error out"=w455:errorcluster, "Receive Log File Path"=w452:path)  [unwired: 8 in]
            n225 = case shown="True" TRUE {
              tunnel: [ADCP_UI_Queue_Manager_Commands."Disable Continuous Tx & Rx" ("command") ADCP_UI_Queue_Manager_Commands."Disable Continuous Receiver" ("command")] -> w477
              frame True {
              }
              frame False {
              }
            }
            n226 = property class="Path"(reference=w460, "Val(Sgnl)"=w457) -> ()  [unwired: 1 in, 2 out]
            n227 = property class="Path"(reference=w453, "Val(Sgnl)"=w452) -> ()  [unwired: 1 in, 2 out]
            n228 = call "ADCP_UI_Queue_Manager.vi"("error in (no error)"=w455, "command"=w477, "ADCU_GUI References"=w462) -> ("error out"=w478:errorcluster)  [unwired: 8 in]
            n229 = Unbundle By Name(w462) -> ("Network Error Status"=w491:refnum<vi>)
            n230 = Bundle By Name(cluster=w490, "Node ID"=w492) -> ()  [unwired: 1 out]
            n231 = call "Connection_Management.vi"("CM Packet In"=w490, "Commands"=Connection_Management_Commands."Open Connection", "Retry interval (ms)"=250, "Number of tries"=u8 10, "error in (no error)"=w478) -> ("CM Params Out"=w483:T15, "Network Error Status"=w486:T17, "error out"=w476:errorcluster)  [unwired: 7 in, 1 out]
            n232 = Unbundle By Name(w483) -> ("Open Conn. ACK"=w482:bool)
            n233 = Select(t=ADCP_UI_Node_Requests."Open Connection ACK" ("Value (Signaling)"), s=w482, f=ADCP_UI_Node_Requests."Timeout") -> (s? t:f=w479:T5)
            n234 = property class="Enum (strict)"(reference=w491, "Value"=w486) -> ()  [unwired: 1 in, 2 out]
            n235 = property class="Enum (strict)"(reference=w484, "Val(Sgnl)"=w479) -> ()  [unwired: 1 in, 2 out]
            n236 = call "ADCP_UI_Queue_Manager.vi"("error in (no error)"=w476, "command"=ADCP_UI_Queue_Manager_Commands."Enable Continuous Tx & Rx", "ADCU_GUI References"=w462) -> ("error out"=w475:errorcluster)  [unwired: 8 in]
          }
          frame False {
            w519 = T7 {"Raw Bytes"=[], "Checksum"=FALSE, "Direction"=enum."Transmit", "Processed Bytes"=[], "Node ID"=0, "Packet type"=enum."Data", "Frame Data"=0, "Priority"=enum."LOW", "Frame ID"=0} ("CM Packet In")
            n237 = Unbundle By Name(w502) -> ("Node names"=w523:refnum<vi>)
            n238 = Unbundle By Name(w502) -> ("Node Requests"=w513:refnum<vi>)
            n239 = property class="CmbBox"(reference=w523) -> ("Value"=w522:string)  [unwired: 1 in, 2 out]
            n240 = flat-sequence {
              tunnel: w514 -> [w528]
              tunnel: [w528] -> w507
              tunnel: w513 -> [w527]
              frame #0 {
                n241 = property class="Enum (strict)"(reference=w527, "Val(Sgnl)"=ADCP_UI_Node_Requests."Close Connection RQST" ("Value (Signaling)")) -> ()  [unwired: 1 in, 2 out]
              }
            }
            n242 = Decimal String To Number(string=w522) -> (number=w521:i32)  [unwired: 2 in, 1 out]
            n243 = case shown="False" TRUE {
              tunnel: [ADCP_UI_Queue_Manager_Commands."Disable Continuous Receiver" ("command") ADCP_UI_Queue_Manager_Commands."Disable Continuous Tx & Rx" ("command")] -> w505
              frame False {
              }
              frame True {
              }
            }
            n244 = call "ADCP_UI_Queue_Manager.vi"("error in (no error)"=w507, "command"=w505, "ADCU_GUI References"=w502) -> ("error out"=w506:errorcluster)  [unwired: 8 in]
            n245 = Unbundle By Name(w502) -> ("Network Error Status"=w520:refnum<vi>)
            n246 = Bundle By Name(cluster=w519, "Node ID"=w521) -> ()  [unwired: 1 out]
            n247 = call "Connection_Management.vi"("CM Packet In"=w519, "Commands"=Connection_Management_Commands."Close Connection", "Retry interval (ms)"=250, "Number of tries"=u8 10, "error in (no error)"=w506) -> ("CM Params Out"=w512:T15, "Network Error Status"=w515:T17, "error out"=w504:errorcluster)  [unwired: 7 in, 1 out]
            n248 = Unbundle By Name(w512) -> ("Close Conn. ACK"=w511:bool)
            n249 = Select(t=ADCP_UI_Node_Requests."Close Connection ACK" ("Value (Signaling)"), s=w511, f=ADCP_UI_Node_Requests."Timeout") -> (s? t:f=w508:T5)
            n250 = property class="Enum (strict)"(reference=w520, "Value"=w515) -> ()  [unwired: 1 in, 2 out]
            n251 = property class="Enum (strict)"(reference=w513, "Val(Sgnl)"=w508) -> ()  [unwired: 1 in, 2 out]
            n252 = call "ADCP_UI_Queue_Manager.vi"("error in (no error)"=w504, "command"=ADCP_UI_Queue_Manager_Commands."Enable Continuous Transmitter", "ADCU_GUI References"=w502) -> ("error out"=w503:errorcluster)  [unwired: 8 in]
          }
        }
      }
      event "Request frames from node": Value Change {
        n253 = event-data() -> ("NewVal"=w533:bool)  [unwired: 1 in, 5 out]
        n254 = case shown="True" w533 {
          tunnel: w532 -> [w556 w614]
          tunnel: [w537 w608] -> w531
          tunnel: w530 -> [w536 w616]
          tunnel: [w536 w616] -> w529
          frame True {
            w566 = u8 10 ("Number of tries")
            w565 = 250 ("Retry interval (ms)")
            w567 = T7 {"Raw Bytes"=[], "Checksum"=FALSE, "Direction"=enum."Transmit", "Processed Bytes"=[], "Node ID"=0, "Packet type"=enum."Data", "Frame Data"=0, "Priority"=enum."LOW", "Frame ID"=0} ("CM Packet In")
            n255 = Unbundle By Name(w536) -> ("Request frames"=w544:refnum<vi>)
            n256 = Unbundle By Name(w536) -> ("Node Requests"=w562:refnum<vi>)
            n257 = Unbundle By Name(w536) -> ("Node names"=w572:refnum<vi>)
            n258 = Unbundle By Name(w536) -> ("Request Frame"=w543:refnum<vi>)
            n259 = call "ADCP_UI_Queue_Manager.vi"("error in (no error)"=w556, "command"=ADCP_UI_Queue_Manager_Commands."Disable Continuous Tx & Rx", "ADCU_GUI References"=w536) -> ("error out"=w555:errorcluster)  [unwired: 8 in]
            n260 = property class="Arr (strict)"(reference=w544) -> ("Value"=w540:string[])  [unwired: 1 in, 2 out]
            n261 = property class="CmbBox"(reference=w572) -> ("Value"=w571:string)  [unwired: 1 in, 2 out]
            n262 = flat-sequence {
              tunnel: w555 -> [w607]
              tunnel: [w607] -> w542
              tunnel: w562 -> [w606]
              frame #0 {
                n263 = property class="Enum (strict)"(reference=w606, "Val(Sgnl)"=ADCP_UI_Node_Requests."Remote Request RQST" ("Value (Signaling)")) -> ()  [unwired: 1 in, 2 out]
              }
            }
            n264 = Decimal String To Number(string=w571) -> (number=w570:i32)  [unwired: 2 in, 1 out]
            n265 = for {
              tunnel: w543 -> [w582]
              tunnel: w542 -> [w580]
              tunnel: [w580] -> w541
              tunnel: w540 -> [w579] mode=indexing
              tunnel: [w573] -> w539 mode=indexing
              n266 = property class="CmbBox"(reference=w582) -> ("Strings And Values[]"=w578:T14)  [unwired: 1 in, 2 out]
              n267 = for {
                tunnel: w578 -> [w584] mode=indexing
                tunnel: [w583] -> w581 mode=indexing
                n268 = Unbundle By Name(w584) -> ("String"=w583:string)
              }
              n269 = Search 1D Array(1D array=w581, element=w579) -> (index of element=w577:i32)  [unwired: 1 in]
              n270 = Index Array(array=w578, index=w577) -> (element=w576:cluster{"String":string, "Value":string})
              n271 = Unbundle By Name(w576) -> ("Value"=w575:string)
              n272 = Decimal String To Number(string=w575) -> (number=w574:i32)  [unwired: 2 in, 1 out]
              n273 = To Unsigned Byte Integer(number=w574) -> (unsigned 8bit integer=w573:u8)
            }
            n274 = Unbundle By Name(w536) -> ("Enable/disable node"=w553:refnum<vi>, "Network Error Status"=w569:refnum<vi>)
            n275 = Bundle By Name(cluster=w567, "Node ID"=w570) -> ()  [unwired: 1 out]
            n276 = call "Remote_Request.vi"("FIDs"=w539, "error in (no error)"=w541, "Retry interval (ms)"=w565, "Number of tries"=w566, "RREQ Packet"=w567) -> ("error out"=w568:errorcluster, "Processed Bytes"=w546:u8[][], "RREQ Param Out"=w561:T18)  [unwired: 3 in, 1 out]
            n277 = Unbundle By Name(w561) -> ("Remote Ack."=w560:bool)
            n278 = call "Error_and_Status.vi"("error in (no error)"=w568, "Retry interval (ms)"=w565, "Number of tries"=w566, "ES Packet"=w567) -> ("error out"=w547:errorcluster, "ES Param Out"=w564:T16)  [unwired: 5 in, 1 out]
            n279 = Unbundle By Name(w564) -> ("Network Error Status"=w563:T17)
            n280 = Select(t=ADCP_UI_Node_Requests."Remote Request ACK" ("Enum"), s=w560, f=ADCP_UI_Node_Requests."Timeout") -> (s? t:f=w557:T5)
            n281 = Matrix Size(0:w546) -> (1:w548:i32)  [unwired: 1 out]
            n282 = for {
              N: w548 -> [_]
              tunnel: w547 -> [w602]
              tunnel: w546 -> [w604]
              tunnel: [w586] -> w545
              i -> [w603]
              n283 = Index Array(array=w604, index (row)=w603) -> (element=w594:u8[])  [unwired: 1 in]
              n284 = call "Processed_To_Raw_Bytes.vi"("Processed Bytes"=w594) -> ("Node ID"=w599:u8, "Raw Bytes"=w598:u8[])  [unwired: 1 in, 3 out]
              n285 = Index Array(array=w598, index=1) -> (element=w596:u8)
              n286 = call "Receiver_Statistics.vi"("error in (no error)"=w602, "Frame ID"=w596, "Node ID"=w599, "Initialize ?"=FALSE) -> ("error out"=w601:errorcluster, "Output"=w595:T19)  [unwired: 5 in, 1 out]
              n287 = Unbundle By Name(w595) -> ("Time interval (ms)"=w592:u32, "Last received time (ms)"=w593:u32, "Count"=w591:u32)
              n288 = call "Update_Data_Packet_From_Processed_Bytes_Receiver.vi"("Processed Bytes"=w594, "Receive count"=w591, "Receive interval (ms)"=w592, "Last Receive Time (ms)"=w593, "error in (no error)"=w601) -> ("Updated data packet"=w589:T20, "error out"=w590:errorcluster)  [unwired: 8 in, 1 out]
              n289 = call "Read_Parameters_From_Data_Packet.vi"("error in (no error)"=w590, "Data_Packet in"=w589) -> ("error out"=w588:errorcluster, "Data Packets Out"=w587:T20[])  [unwired: 7 in, 1 out]
              n290 = call "Data_Packets_To_Receiver_Table_Formatter.vi"("error in (no error)"=w588, "Data Packets In"=w587) -> ("error out"=w586:errorcluster, "Table contents"=w585:string[][])  [unwired: 8 in]
              n291 = global write "ADCP_UI_Receive_List_Data_Packets.vi" "Receive List Table Contents"(w585) -> ()
            }
            n292 = property class="Enum (strict)"(reference=w569, "Value"=w563) -> ()  [unwired: 1 in, 2 out]
            n293 = property class="Enum (strict)"(reference=w562, "Val(Sgnl)"=w557) -> ()  [unwired: 1 in, 2 out]
            n294 = property class="Bool (strict)"(reference=w553) -> ("Value"=w552:bool)  [unwired: 1 in, 2 out]
            n295 = Select(t=ADCP_UI_Queue_Manager_Commands."Enable Continuous Receiver" ("command"), s=w552, f=ADCP_UI_Queue_Manager_Commands."Disable Continuous Receiver" ("command")) -> (s? t:f=w549:T4)
            n296 = call "ADCP_UI_Queue_Manager.vi"("error in (no error)"=w545, "command"=w549, "ADCU_GUI References"=w536) -> ("error out"=w538:errorcluster)  [unwired: 8 in]
            n297 = call "ADCP_UI_Queue_Manager.vi"("error in (no error)"=w538, "command"=ADCP_UI_Queue_Manager_Commands."Enable Continuous Transmitter", "ADCU_GUI References"=w536) -> ("error out"=w537:errorcluster)  [unwired: 8 in]
          }
          frame False {
            w615 = T7 {"Raw Bytes"=[], "Checksum"=FALSE, "Direction"=enum."Transmit", "Processed Bytes"=[], "Node ID"=0, "Packet type"=enum."Data", "Frame Data"=0, "Priority"=enum."LOW", "Frame ID"=0} ("CM Packet In")
            n298 = Unbundle By Name(w616) -> ("Node names"=w620:refnum<vi>)
            n299 = property class="CmbBox"(reference=w620) -> ("Value"=w619:string)  [unwired: 1 in, 2 out]
            n300 = Decimal String To Number(string=w619) -> (number=w618:i32)  [unwired: 2 in, 1 out]
            n301 = Unbundle By Name(w616) -> ("Network Error Status"=w617:refnum<vi>)
            n302 = Bundle By Name(cluster=w615, "Node ID"=w618) -> ()  [unwired: 1 out]
            n303 = call "Connection_Management.vi"("CM Packet In"=w615, "Commands"=Connection_Management_Commands."Close Connection", "Retry interval (ms)"=250, "Number of tries"=u8 10, "error in (no error)"=w614) -> ("CM Params Out"=w609:T15, "Network Error Status"=w610:T17, "error out"=w608:errorcluster)  [unwired: 7 in, 1 out]
            n304 = flat-sequence {
              tunnel: w609 -> [_]
              frame #0 {
              }
            }
            n305 = property class="Enum (strict)"(reference=w617, "Value"=w610) -> ()  [unwired: 1 in, 2 out]
          }
        }
      }
      event "Add transmit list frame": Value Change {
        n306 = event-data() -> ("NewVal"=w624:bool)  [unwired: 1 in, 5 out]
        n307 = case shown="True" w624 {
          tunnel: w625 -> [w628 w654]
          tunnel: [w628 w634] -> w623
          tunnel: w622 -> [w627 w658]
          tunnel: [w627 w658] -> w621
          frame False {
          }
          frame True {
            n308 = Unbundle By Name(w658) -> ("Transmit List Frame name"=w659:refnum<vi>)
            n309 = Unbundle By Name(w658) -> ("Node names"=w657:refnum<vi>)
            n310 = Unbundle By Name(w658) -> ("Transmit List"=w660:refnum<vi>)
            n311 = property class="Tbl (strict)"(reference=w660) -> (reference out=w631:refnum<vi>, "Value"=w641:string[][])  [unwired: 1 in, 1 out]
            n312 = property class="CmbBox"(reference=w659) -> ("Value"=w656:string)  [unwired: 1 in, 2 out]
            n313 = property class="CmbBox"(reference=w657) -> ("Value"=w655:string)  [unwired: 1 in, 2 out]
            n314 = Decimal String To Number(string=w656) -> (number=w651:i32)  [unwired: 2 in, 1 out]
            n315 = Decimal String To Number(string=w655) -> (number=w652:i32)  [unwired: 2 in, 1 out]
            n316 = call "Data_Packet_FGV.vi"("Node ID"=w652, "Frame ID"=w651, "error in (no error)"=w654, "Commands"=Data_Packet_FGV_Commands."Read Data Packet from Node ID and Frame ID") -> ("Data_Packet out"=w637:T20, "error out"=w639:errorcluster)  [unwired: 6 in, 4 out]
            n317 = Index Array(array=w641, index (col)=0 ("disabled index (col)")) -> (element=w649:string[])  [unwired: 1 in]
            n318 = Bundle By Name(cluster=w637, "Transmit count"=-1, "Transmit_Mode"=Data_Packet_Transmit_Mode."Disabled", "Transmit Enable"=FALSE) -> (w629:T20)
            n319 = Unbundle By Name(w637) -> ("Parameters"=w648:T12[])
            n320 = call "Data_Packet_FGV.vi"("Data_Packet In"=w629, "error in (no error)"=w639, "Commands"=Data_Packet_FGV_Commands."Update Packet") -> ("Data Packets Out"=w635:T20[], "error out"=w638:errorcluster)  [unwired: 7 in, 4 out]
            n321 = Index Array(array=w648, index=0) -> (element=w646:T12)
            n322 = Unbundle By Name(w646) -> ("Node name"=w645:string, "Frame name"=w644:string)
            n323 = Concatenate Strings(w645, ":" ("string"), w644) -> (w642:string)
            n324 = for {
              tunnel: w649 -> [w665] mode=indexing
              tunnel: w642 -> [w664]
              tunnel: [w661] -> _
              stop <- w661 stop-if-true
              n325 = Search and Replace String(input string=w665, search string=w664) -> (number of replacements=w663:i32)  [unwired: 6 in, 3 out]
              n326 = Not Equal?(x=w663, y=0) -> (x != y?=w661:bool)
            }
            n327 = call "Data_Packets_To_Transmitter_Table_Formatter.vi"("error in (no error)"=w638, "Data Packets In"=w635) -> ("error out"=w634:errorcluster, "Table contents"=w630:string[][])  [unwired: 8 in]
            n328 = property class="Tbl (strict)"(reference=w631, "Value"=w630) -> ()  [unwired: 1 in, 2 out]
          }
        }
      }
      event "Remove transmit list frame": Value Change {
        n329 = event-data() -> ("NewVal"=w669:bool)  [unwired: 1 in, 5 out]
        n330 = case shown="True" w669 {
          tunnel: w670 -> [w673 w699]
          tunnel: [w673 w679] -> w668
          tunnel: w667 -> [w672 w703]
          tunnel: [w672 w703] -> w666
          frame False {
          }
          frame True {
            n331 = Unbundle By Name(w703) -> ("Transmit List Frame name"=w704:refnum<vi>)
            n332 = Unbundle By Name(w703) -> ("Node names"=w702:refnum<vi>)
            n333 = Unbundle By Name(w703) -> ("Transmit List"=w705:refnum<vi>)
            n334 = property class="Tbl (strict)"(reference=w705) -> (reference out=w676:refnum<vi>, "Value"=w686:string[][])  [unwired: 1 in, 1 out]
            n335 = property class="CmbBox"(reference=w704) -> ("Value"=w701:string)  [unwired: 1 in, 2 out]
            n336 = property class="CmbBox"(reference=w702) -> ("Value"=w700:string)  [unwired: 1 in, 2 out]
            n337 = Decimal String To Number(string=w701) -> (number=w696:i32)  [unwired: 2 in, 1 out]
            n338 = Decimal String To Number(string=w700) -> (number=w697:i32)  [unwired: 2 in, 1 out]
            n339 = call "Data_Packet_FGV.vi"("Node ID"=w697, "Frame ID"=w696, "error in (no error)"=w699, "Commands"=Data_Packet_FGV_Commands."Read Data Packet from Node ID and Frame ID") -> ("Data_Packet out"=w682:T20, "error out"=w684:errorcluster)  [unwired: 6 in, 4 out]
            n340 = Index Array(array=w686, index (col)=0 ("disabled index (col)")) -> (element=w694:string[])  [unwired: 1 in]
            n341 = Bundle By Name(cluster=w682, "Transmit count"=-2, "Transmit_Mode"=Data_Packet_Transmit_Mode."Disabled", "Transmit Enable"=FALSE) -> (w674:T20)
            n342 = Unbundle By Name(w682) -> ("Parameters"=w693:T12[])
            n343 = call "Data_Packet_FGV.vi"("Data_Packet In"=w674, "error in (no error)"=w684, "Commands"=Data_Packet_FGV_Commands."Update Packet") -> ("Data Packets Out"=w680:T20[], "error out"=w683:errorcluster)  [unwired: 7 in, 4 out]
            n344 = Index Array(array=w693, index=0) -> (element=w691:T12)
            n345 = Unbundle By Name(w691) -> ("Node name"=w690:string, "Frame name"=w689:string)
            n346 = Concatenate Strings(w690, ":" ("string"), w689) -> (w687:string)
            n347 = for {
              tunnel: w694 -> [w710] mode=indexing
              tunnel: w687 -> [w709]
              tunnel: [w706] -> _
              stop <- w706 stop-if-true
              n348 = Search and Replace String(input string=w710, search string=w709) -> (number of replacements=w708:i32)  [unwired: 6 in, 3 out]
              n349 = Not Equal?(x=w708, y=0) -> (x != y?=w706:bool)
            }
            n350 = call "Data_Packets_To_Transmitter_Table_Formatter.vi"("error in (no error)"=w683, "Data Packets In"=w680) -> ("error out"=w679:errorcluster, "Table contents"=w675:string[][])  [unwired: 8 in]
            n351 = property class="Tbl (strict)"(reference=w676, "Value"=w675) -> ()  [unwired: 1 in, 2 out]
          }
        }
      }
    }
  }
